vi "save HAS file as png with scaling txt file.vi"(8 "error in (no error)":errorcluster, 10 "configuration file path":path, 11 "Mean wavefront":dbl[][](graph)) -> (0 "error out 2":errorcluster)   [LabVIEW 2020]
uses:
  <vilib>/Utility/config.llb/Write Key (Double).vi
  <vilib>/Utility/config.llb/NI_LVConfig.lvlib
panel:
  out "Mean wavefront 2":dbl[][](graph)
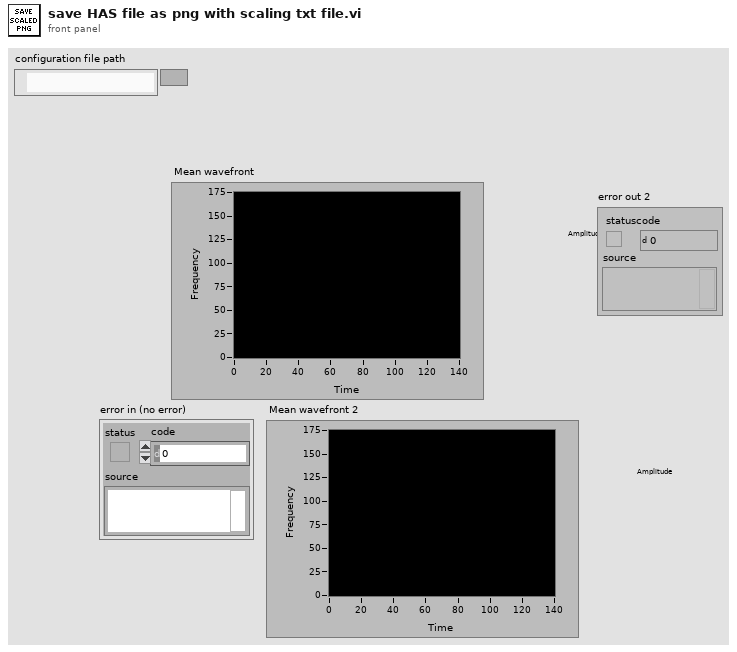
[diagram p1: front panel]
types:
  T1 = typedef "Image Type" = u32
  T2 = typedef "NI_LVConfig.lvlib/Config Data RefNum.ctl" = refnum<k1>
  T3 = typedef "IMAQ Image.ctl" = refnum<image>
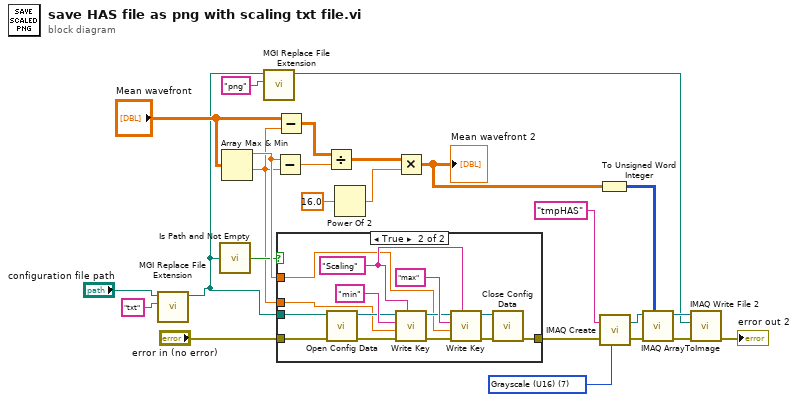
[diagram p0: block diagram]
diagram:
  w14 = T1 7 items=["Grayscale (U8)", "Grayscale (I16)", "Grayscale (SGL)", "Complex (CSG)", "RGB (U32)", "HSL (U32)", "RGB (U64)", "Grayscale (U16)"] ("Image Type")
  n1 = call "MGI Replace File Extension.vi"("New Extension (txt)"="txt", "Path In"="configuration file path") -> ("Path Out"=w1:path)  [unwired: 8 in, 1 out]
  n2 = call <vilib>:"Is Path and Not Empty.vi"("path"=w1) -> ("Is Path and Not Empty?"=w22:bool)  [unwired: 4 in]
  n3 = Array Max & Min(array="Mean wavefront") -> (max value=w24:dbl, min value=w17:dbl)  [unwired: 2 out]
  n4 = call "MGI Replace File Extension.vi"("New Extension (txt)"="png", "Path In"=w1) -> ("Path Out"=w8:path)  [unwired: 8 in, 1 out]
  n5 = Subtract(x=w24, y=w17) -> (x-y=w21:dbl)
  n6 = Subtract(x="Mean wavefront", y=w17) -> (x-y=w16:dbl[][])
  n7 = case shown="True" w22 {
    tunnel: "error in (no error)" -> [w26 w31]
    tunnel: w24 -> [_ w30]
    tunnel: w17 -> [_ w29]
    tunnel: w1 -> [_ w28]
    tunnel: [w26 w27] -> w4
    frame False {
    }
    frame True {
      w37 = "Scaling" ("section")
      n8 = call <vilib>:"Open Config Data.vi"("error in (no error)"=w31, "configuration file path"=w28) -> ("error out"=w34:errorcluster, "refnum"=w39:T2)  [unwired: 7 in, 1 out]
      n9 = call-poly <vilib>:"Write Key.vi"("section"=w37, "error in (no error)"=w34, "value"=w29, "key"="min", "refnum"=w39) -> ("error out"=w33:errorcluster, "refnum out"=w36:T2)  [unwired: 4 in, 1 out]
      n10 = call-poly <vilib>:"Write Key.vi"("section"=w37, "error in (no error)"=w33, "value"=w30, "key"="max", "refnum"=w36) -> ("error out"=w32:errorcluster, "refnum out"=w35:T2)  [unwired: 4 in, 1 out]
      n11 = call <vilib>:"Close Config Data.vi"("error in (no error)"=w32, "refnum"=w35) -> ("error out"=w27:errorcluster)  [unwired: 8 in, 1 out]
    }
  }
  n12 = Divide(x=w16, y=w21) -> (x/y=w20:dbl[][])
  n13 = Power Of 2(x=16.0) -> (2^x=w19:dbl)
  n14 = Multiply(x=w20, y=w19) -> (x*y=w13:dbl[][])
  "Mean wavefront 2" <- w13
  n15 = To Unsigned Word Integer(number=w13) -> (unsigned 16bit integer=w12:u16[][])
  n16 = call "IMAQ Create"("Image Name"="tmpHAS", "Image Type"=w14, "error in (no error)"=w4) -> ("New Image"=w11:T3, "error out"=w7:errorcluster)  [unwired: 2 in]
  n17 = call "IMAQ ArrayToImage"("Image Pixels (U16)"=w12, "error in (no error)"=w7, "Image"=w11) -> ("error out"=w5:errorcluster, "Image Out"=w10:T3)  [unwired: 7 in]
  n18 = call-poly "IMAQ Write File 2"("error in (no error)"=w5, "File Path"=w8, "Image"=w10) -> ("error out"=→"error out 2":errorcluster)  [unwired: 7 in, 1 out]
